vi "Test Compare Equal 1el String Arrays.vi"(8 "error in (no error)":errorcluster, 11 "Comparison Test Double in":refnum<class "Comparison Test Double.lvclass">) -> (0 "error out":errorcluster, 3 "Comparison Test Double out":refnum<class "Comparison Test Double.lvclass">)   [LabVIEW 2020, in "Comparison Test Double.lvclass"]
uses:
  Comparison Test Double.lvclass
  Comparison Test Double.lvclass/Comparison Test Double.ctl
  2e376786-aa96-4976-8152-b36927c13d03.vi
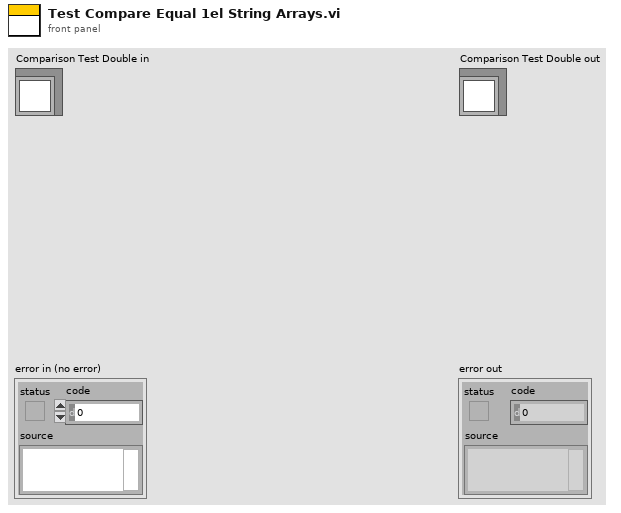
[diagram p1: front panel]
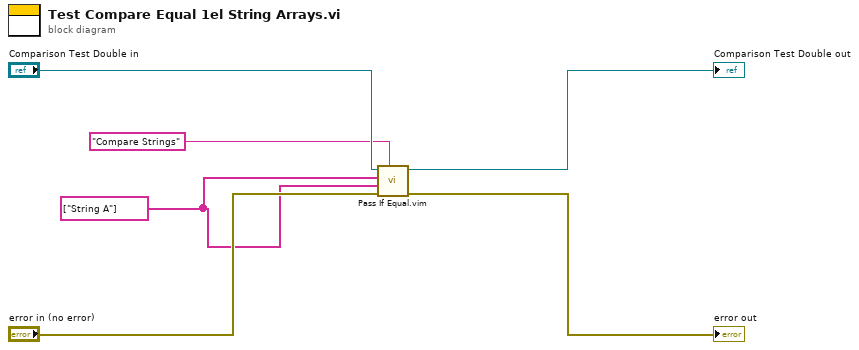
[diagram p0: block diagram]
diagram:
  w1 = string[] ["String A"]
  n1 = call "Pass If Equal.vim"("Description"="Compare Strings", "error in (no error)"="error in (no error)", "Actual"=w1, "Expected"=w1, "LUnit Test Case In"="Comparison Test Double in") -> ("error out"=→"error out":errorcluster, "LUnit Test Case Out"=→"Comparison Test Double out":refnum<class "Comparison Test Double.lvclass">)  [unwired: 5 in]
